vi "Mouse_queue.vi"(7 "Refs cluster In":T1) -> ()   [LabVIEW 2015]
uses:
  <vilib>/Utility/inputDevices.llb/mouseAcquire.vi
  <vilib>/Utility/inputDevices.llb/closeMouse.vi
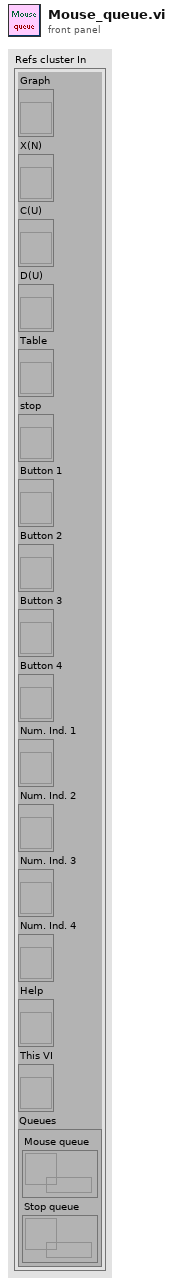
[diagram p1: front panel]
types:
  T1 = cluster{"Graph":refnum<vi>, "X(N)":refnum<vi>, "C(U)":refnum<vi>, "D(U)":refnum<vi>, "Table":refnum<vi>, "stop":refnum<vi>, "Button 1":refnum<vi>, "Button 2":refnum<vi>, "Button 3":refnum<vi>, "Button 4":refnum<vi>, "Num. Ind. 1":refnum<vi>, "Num. Ind. 2":refnum<vi>, "Num. Ind. 3":refnum<vi>, "Num. Ind. 4":refnum<vi>, "Help":refnum<vi>, "This VI":refnum<vi>, "Queues":cluster{"Mouse queue":refnum<queue>, "Stop queue":refnum<queue>}}
  T2 = cluster{"Horizontal":i32, "Vertical":i32, "Scrolling":i32}
  T3 = cluster{"button 1":bool, "button 2":bool, "button 3":bool, "button 4":bool}
  T4 = cluster{"device ID":refnum<k1>, "axis info":cluster{"Horizontal":i32, "Vertical":i32, "Scrolling":i32}, "button info":cluster{"button 1":bool, "button 2":bool, "button 3":bool, "button 4":bool}}
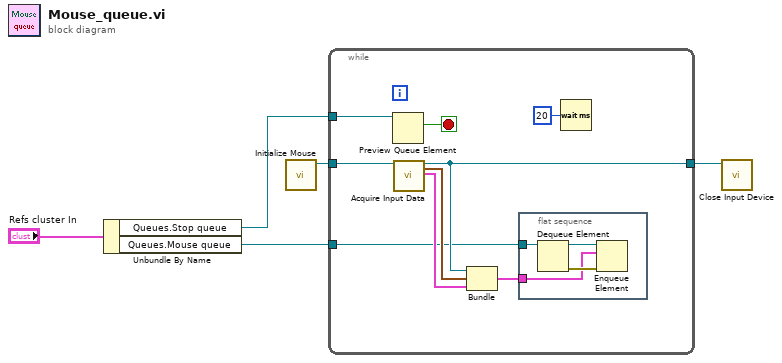
[diagram p0: block diagram]
diagram:
  n1 = Unbundle By Name("Refs cluster In") -> ("Queues.Stop queue"=w2:refnum<queue>, "Queues.Mouse queue"=w1:refnum<queue>)
  n2 = call <vilib>:"Initialize Mouse.vi"() -> ("device ID"=w4:refnum<k1>)  [unwired: 10 in, 1 out]
  n3 = while {
    tunnel: w4 -> [w14]
    tunnel: w2 -> [w9]
    tunnel: [w7] -> w5
    tunnel: w1 -> [w6]
    stop <- w8 stop-if-true
    n4 = Preview Queue Element(queue=w9) -> (element=w8:bool)  [unwired: 2 in, 3 out]
    n5 = call-poly <vilib>:"Acquire Input Data.vi"("device ID"=w14) -> ("device ID"=w7:refnum<k1>, "axis info"=w10:T2, "button info"=w11:T3)  [unwired: 15 in, 1 out]
    n6 = Bundle("device ID"=w7, "axis info"=w10, "button info"=w11) -> (w12:T4)  [unwired: 1 in]
    n7 = flat-sequence {
      tunnel: w12 -> [w17]
      tunnel: w6 -> [w15]
      frame #0 {
        n8 = Dequeue Element(queue=w15) -> (queue out=w16:refnum<queue>, error out=w18:errorcluster)  [unwired: 2 in, 2 out]
        n9 = Enqueue Element(queue=w16, element=w17, error in (no error)=w18) -> ()  [unwired: 1 in, 3 out]
      }
    }
    n10 = Wait (ms)(milliseconds to wait=u32 20) -> ()  [unwired: 1 out]
  }
  n11 = call-poly <vilib>:"Close Input Device.vi"("device ID"=w5) -> ()  [unwired: 9 in, 1 out]
